vi "Init.vi"(8 "error in (no error)":errorcluster, 10 "Channel Count (16)":i32=16, 11 "Audio Device":T1) -> (0 "error out":errorcluster, 3 "Mixer out":refnum<class "Mixer.lvclass">)   [LabVIEW 2020, in "G-Audio.lvlib" / "Mixer.lvclass"]
uses:
  Mixer.lvclass
  Controls/Audio Device Refnum.ctl
  Message.ctl
  Command.ctl
  Mixer.lvclass/Mixer.ctl
  Channel/Channel.lvclass
  G-Audio.lvlib
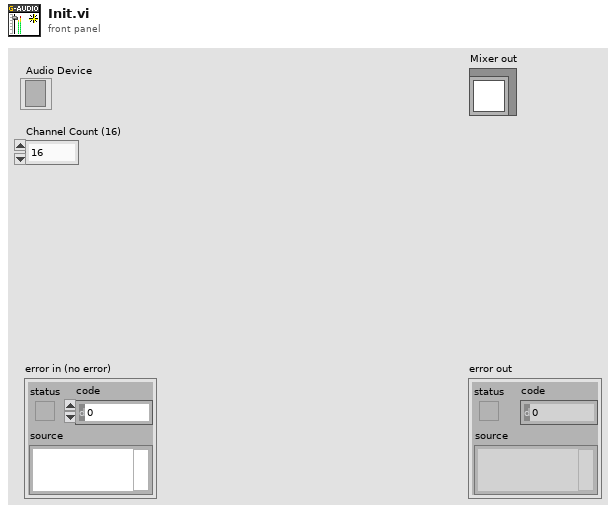
[diagram p1: front panel]
types:
  T1 = typedef "G-Audio.lvlib/Audio Device Refnum.ctl" = refnum<file>
  T2 = typedef "G-Audio.lvlib/Mixer.lvclass/Message.ctl" = cluster{"Command":T3, "Channel":i32, "Payload":variant}
  T3 = typedef "G-Audio.lvlib/Mixer.lvclass/Command.ctl" = enum16{"Channel Stop", "Channel Pause", "Channel Play", "Channel Volume"}
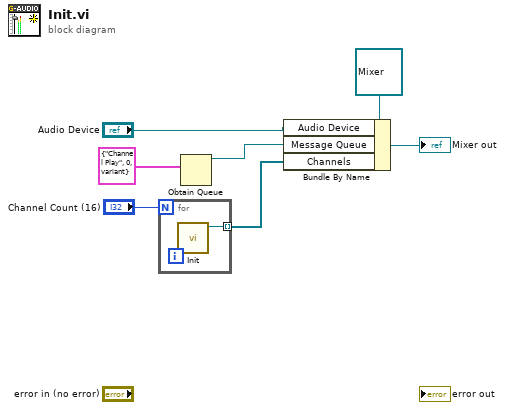
[diagram p0: block diagram]
diagram:
  n1 = for {
    N: "Channel Count (16)" -> [_]
    tunnel: [w8] -> w3 mode=indexing
    n2 = call "Init.vi"() -> ("Channel DVR"=w8:refnum<data-value>)  [unwired: 10 in, 1 out]
  }
  n3 = Obtain Queue(element data type=T2 {"Command"=enum."Channel Play", "Channel"=0, "Payload"=variant} ("Message")) -> (queue out=w5:refnum<queue>)  [unwired: 4 in, 2 out]
  n4 = Bundle By Name(cluster=refnum<class "Mixer.lvclass"> refnum ("Mixer out"), "Audio Device"="Audio Device", "Message Queue"=w5, "Channels"=w3) -> (→"Mixer out":refnum<class "Mixer.lvclass">)
